vi "Restart.CheckValidSelection.vi"(8 "error in (no error)":errorcluster, 10 "Restart Path":path, 11 "State Variables":T1) -> (0 "error out":errorcluster, 2 "Load Restart?":bool, 3 "State Variables out":T1)   [LabVIEW 2013, in "Simple Sequence Tools - Execution.lvlib"]
uses:
  Simple Sequence Tools - Execution.lvlib
  Types/Main.StateVariables.ctl
  Types/Execute.UserEventRefs.ctl
  <vilib>/NI Veristand/Execution/Workspace/SystemStateRegEventRef.ctl
  Types/Execution.SequenceState.ctl
  <vilib>/NI Veristand/Execution/DataLogging/DataLoggingSpecification Ref.ctl
  NationalInstruments.VeriStand.ClientAPI
  <vilib>/NI Veristand/Execution/DataLogging/IDataLogging Ref.ctl
  <vilib>/NI Veristand/Execution/Workspace/WorkspaceAPI.ctl
  NationalInstruments.VeriStand.RealTimeSequenceDefinitionApi
  <vilib>/NI Veristand/Execution/Workspace/SystemStateEventRef.ctl
  Shared/Types/INI.Settings
  Shared/Simple Sequence Tools - Shared.lvlib
  <vilib>/NI Veristand/Execution/Workspace/NI_VS Workspace ExecutionAPI.lvlib
  <vilib>/NI Veristand/Execution/DataLogging/NI_VS Data Logging API.lvlib
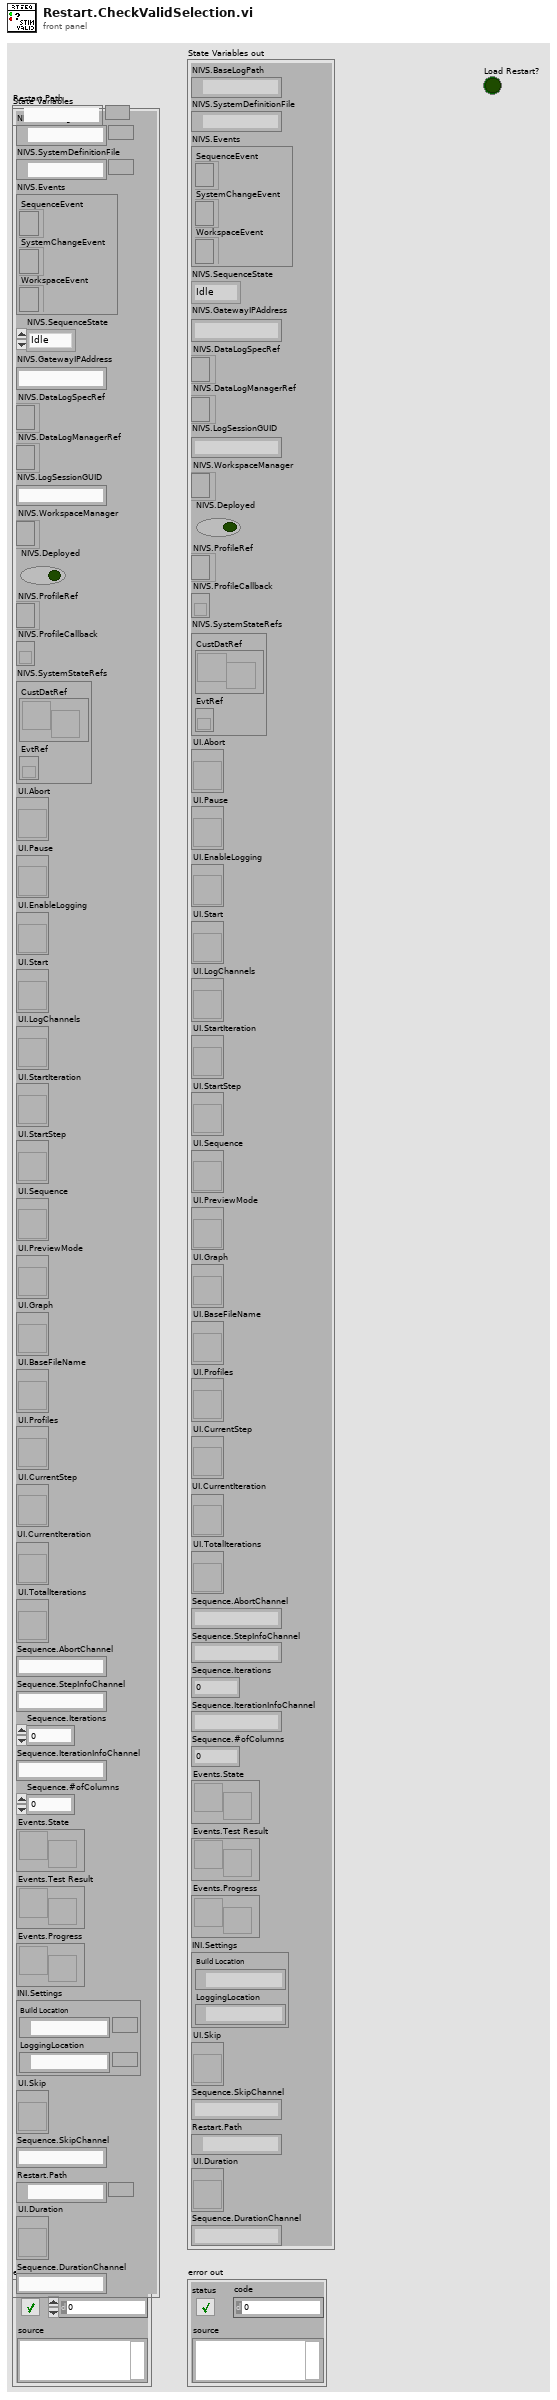
[diagram p1: front panel]
types:
  T1 = typedef "Simple Sequence Tools - Execution.lvlib/Main.StateVariables.ctl" = cluster{"NIVS.BaseLogPath":path, "NIVS.SystemDefinitionFile":path, "NIVS.Events":T2, "NIVS.SequenceState":T4, "NIVS.GatewayIPAddress":string, "NIVS.DataLogSpecRef":T5, "NIVS.DataLogManagerRef":T6, "NIVS.LogSessionGUID":string, "NIVS.WorkspaceManager":T7, "NIVS.Deployed":bool, "NIVS.ProfileRef":refnum<k24>, "NIVS.ProfileCallback":refnum<k27>, "NIVS.SystemStateRefs":T8, "UI.Abort":refnum<vi>, "UI.Pause":refnum<vi>, "UI.EnableLogging":refnum<vi>, "UI.Start":refnum<vi>, "UI.LogChannels":refnum<vi>, "UI.StartIteration":refnum<vi>, "UI.StartStep":refnum<vi>, "UI.Sequence":refnum<vi>, "UI.PreviewMode":refnum<vi>, "UI.Graph":refnum<vi>, "UI.BaseFileName":refnum<vi>, "UI.Profiles":refnum<vi>, "UI.CurrentStep":refnum<vi>, "UI.CurrentIteration":refnum<vi>, "UI.TotalIterations":refnum<vi>, "Sequence.AbortChannel":string, "Sequence.StepInfoChannel":string, "Sequence.Iterations":u32, "Sequence.IterationInfoChannel":string, "Sequence.#ofColumns":i32, "Events.State":refnum<user-event>, "Events.Test Result":refnum<user-event>, "Events.Progress":refnum<user-event>, "INI.Settings":T9, "UI.Skip":refnum<vi>, "Sequence.SkipChannel":string, "Restart.Path":path, "UI.Duration":refnum<vi>, "Sequence.DurationChannel":string}
  T2 = typedef "Simple Sequence Tools - Execution.lvlib/Execute.UserEventRefs.ctl" = cluster{"SequenceEvent":refnum<event-registration>, "SystemChangeEvent":T3, "WorkspaceEvent":refnum<event-registration>}
  T3 = typedef "NI_VS Workspace ExecutionAPI.lvlib/SystemStateRegEventRef.ctl" = refnum<event-registration>
  T4 = typedef "Simple Sequence Tools - Execution.lvlib/Execution.SequenceState.ctl" = enum16{"Idle", "Initializing", "Running", "Paused", "Finalizing", "Complete"}
  T5 = typedef "NI_VS Data Logging API.lvlib/DataLoggingSpecification Ref.ctl" = refnum<k24>
  T6 = typedef "NI_VS Data Logging API.lvlib/IDataLogging Ref.ctl" = refnum<k24>
  T7 = typedef "NI_VS Workspace ExecutionAPI.lvlib/WorkspaceAPI.ctl" = refnum<k24>
  T8 = typedef "NI_VS Workspace ExecutionAPI.lvlib/SystemStateEventRef.ctl" = cluster{"CustDatRef":refnum<user-event>, "EvtRef":refnum<k27>}
  T9 = typedef "Simple Sequence Tools - Shared.lvlib/INI.Settings" = cluster{"Build Location":path, "LoggingLocation":path}
  T10 = typedef "Simple Sequence Tools - Execution.lvlib/Restart.Settings" = cluster{"LogFile":path, "Log Settings":T11[], "StimulusProfile":path, "StopIteration":u32, "StopStep":u32, "Log Channels":T15, "Base File Name":string, "Enable Logging":bool, "Profile":string, "StopDuration":dbl}
  T11 = typedef "NI_VS Data Logging API.lvlib/TDMS Channel Group.ctl" = cluster{"Group Name":string, "Group Description":string, "Group Properties":T12[], "Channels":T13[], "Time Channel Options":T14, "Time Channel Name":string}
  T12 = typedef "NI_VS Data Logging API.lvlib/TDMS Property.ctl" = cluster{"Name":string, "Value":variant}
  T13 = typedef "NI_VS Data Logging API.lvlib/TDMS Channel.ctl" = cluster{"Channel Name":string, "Channel Path":string, "Channel Description":string, "Channel Properties":T12[]}
  T14 = typedef "NI_VS Data Logging API.lvlib/Time Channel Options.ctl" = enum16{"No Time Channel", "Absolute Time", "System Time", "System Time - Microseconds", "Absolute Time as Double"}
  T15 = typedef "Simple Sequence Tools - Execution.lvlib/Log.SelectedChannels.ctl" = enum16{"Channels (No System Channel)", "Aliases", "All"}
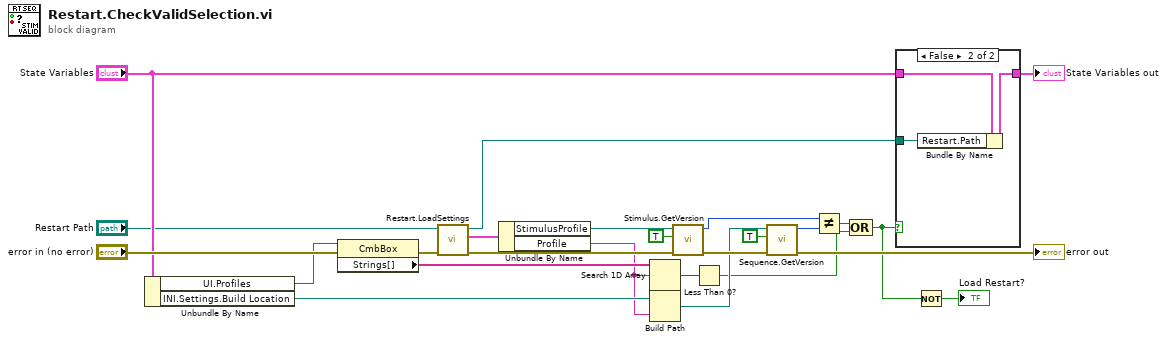
[diagram p0: block diagram]
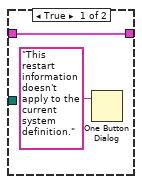
[diagram p2: hidden frame]
diagram:
  n1 = Unbundle By Name("State Variables") -> ("UI.Profiles"=w21:refnum<vi>, "INI.Settings.Build Location"=w11:path)
  n2 = property class="CmbBox"(reference=w21, error in="error in (no error)") -> (error out=w23:errorcluster, "Strings[]"=w24:string[])  [unwired: 1 out]
  n3 = call "Restart.LoadSettings.vi"("error in"=w23, "path (use dialog)"="Restart Path") -> ("error out"=w8:errorcluster, "Restart Settings"=w19:T10, "path"=w18:path)  [unwired: 7 in]
  n4 = Unbundle By Name(w19) -> ("StimulusProfile"=w9:path, "Profile"=w4:string)
  n5 = Search 1D Array(1D array=w24, element=w4) -> (index of element=w25:i32)  [unwired: 1 in]
  n6 = Build Path(base path=w11, name or relative path=w4) -> (appended path=w10:path)
  n7 = call "Stimulus.GetVersion.vi"("error in (no error)"=w8, "Exists"=TRUE, "Path"=w9) -> ("error out"=w14:errorcluster, "Build"=w12:u32)  [unwired: 7 in]
  n8 = Less Than 0?(x=w25) -> (x < 0?=w5:bool)
  n9 = call "Sequence.GetVersion.vi"("error in (no error)"=w14, "Exists"=TRUE, "Path"=w10) -> ("error out"=→"error out":errorcluster, "Build"=w13:u32)  [unwired: 7 in]
  n10 = Not Equal?(x=w12, y=w13) -> (x != y?=w6:bool)
  n11 = Compound Arithmetic op=OR(w6, w5) -> (w3:bool)
  n12 = case shown="False" w3 {
    tunnel: [w27 w30] -> w16
    tunnel: w18 -> [_ w29]
    tunnel: "State Variables" -> [w27 w28]
    frame True {
      n13 = One Button Dialog(message="This restart information doesn't apply to the current system definition.") -> ()  [unwired: 1 in, 1 out]
    }
    frame False {
      n14 = Bundle By Name(cluster=w28, "Restart.Path"=w29) -> (w30:T1)
    }
  }
  "State Variables out" <- w16
  n15 = Not(x=w3) -> (.not. x?=→"Load Restart?":bool)
